vi "toml_api_resolve_name.vi"(1 "name":string) -> (0 "resolved name":string)   [LabVIEW 2017]
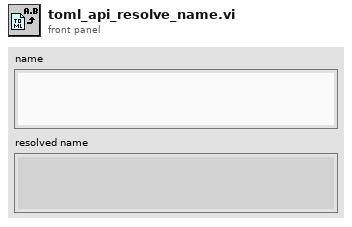
[diagram p1: front panel]
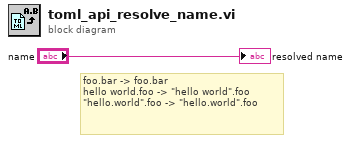
[diagram p0: block diagram]
diagram:
  # "foo.bar -> foo.bar\nhello world.foo -> \"hello world\".foo\n\"hello.world\".foo -> \"hello.world\".foo"
  "resolved name" <- "name"
